vi "tessst.vi"   [LabVIEW 2013]
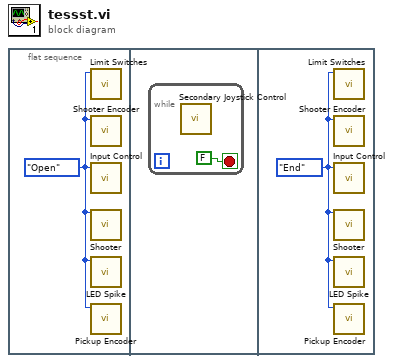
[diagram p0: block diagram]
diagram:
  n1 = flat-sequence {
    frame #0 {
      w1 = enum16{"Open", "Run", "End"}."Open" ("State Control")
      n2 = call "Limit Switches.vi"("State Control"=w1) -> ()  [unwired: 7 in, 4 out]
      n3 = call "Shooter Encoder.vi"("State Control"=w1) -> ()  [unwired: 3 in, 4 out]
      n4 = call "Input Control.vi"("State"=w1) -> ()  [unwired: 2 in, 3 out]
      n5 = call "Shooter.vi"("State Control"=w1) -> ()  [unwired: 17 in, 2 out]
      n6 = call "LED Spike.vi"("State"=w1) -> ()  [unwired: 11 in]
      n7 = call "Pickup Encoder.vi"("State Control"=w1) -> ()  [unwired: 3 in, 4 out]
    }
    frame #1 {
      n8 = while {
        stop <- FALSE stop-if-true
        n9 = call "Secondary Joystick Control.vi"() -> ()  [unwired: 12 in]
      }
    }
    frame #2 {
      w3 = enum16{"Open", "Run", "End"}."End" ("State Control")
      n10 = call "Limit Switches.vi"("State Control"=w3) -> ()  [unwired: 7 in, 4 out]
      n11 = call "Shooter Encoder.vi"("State Control"=w3) -> ()  [unwired: 3 in, 4 out]
      n12 = call "Input Control.vi"("State"=w3) -> ()  [unwired: 2 in, 3 out]
      n13 = call "Shooter.vi"("State Control"=w3) -> ()  [unwired: 17 in, 2 out]
      n14 = call "LED Spike.vi"("State"=w3) -> ()  [unwired: 11 in]
      n15 = call "Pickup Encoder.vi"("State Control"=w3) -> ()  [unwired: 3 in, 4 out]
    }
  }
